vi "Write Fetch Type.vi"(8 "error in (no error)":errorcluster, 10 "Fetch Type":string, 11 "Skyworks - PVT in":refnum<class "Skyworks - PVT.lvclass">) -> (0 "error out":errorcluster, 3 "Skyworks - PVT out":refnum<class "Skyworks - PVT.lvclass">)   [LabVIEW 2018, in "Skyworks PVT.lvlib" / "Skyworks - PVT.lvclass"]
uses:
  Skyworks - PVT.lvclass
  Skyworks - PVT.lvclass/Skyworks - PVT.ctl
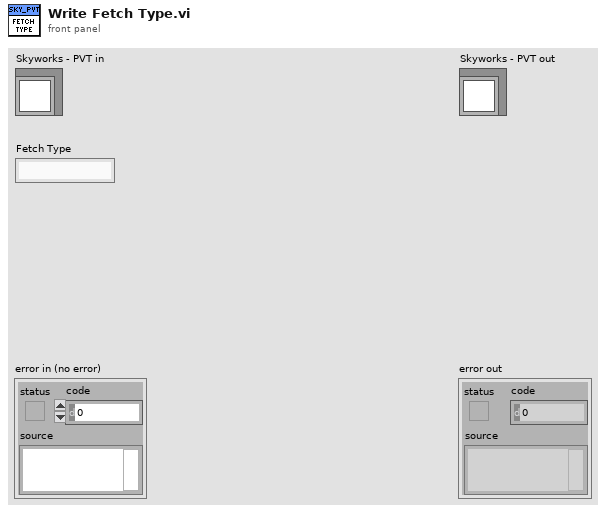
[diagram p1: front panel]
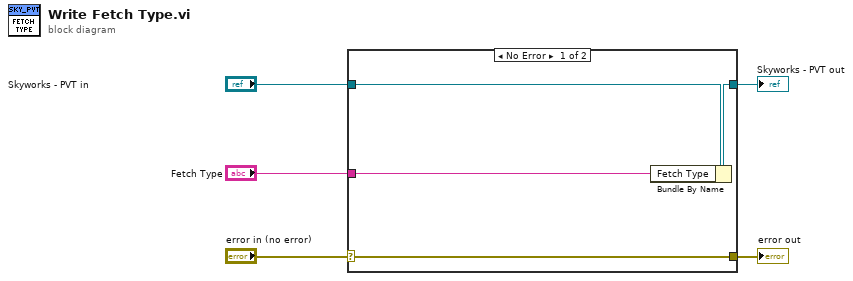
[diagram p0: block diagram]
diagram:
  n1 = case shown="No Error" "error in (no error)" {
    selector: "error in (no error)" -> [w9 w10]
    tunnel: [w9 w10] -> w4
    tunnel: [w7 w11] -> w2
    tunnel: "Skyworks - PVT in" -> [w8 w11]
    tunnel: "Fetch Type" -> [w6 _]
    frame No Error {
      n2 = Bundle By Name(cluster=w8, "Fetch Type"=w6) -> (w7:refnum<class "Skyworks - PVT.lvclass">)
    }
    frame Error {
    }
  }
  "error out" <- w4
  "Skyworks - PVT out" <- w2
